vi "FolderMon Garbage Collector.vi"   [LabVIEW 2011]
uses:
  ITK EXT/utils/strutil.llb/Case Matching.ctl
  Summitek EXT/OpenG EXT/file/file.llb/File Exists - Scalar__ogtk.vi
  server lib/Spartan CONFIG Global.vi
types:
  T1 = typedef "Case Matching.ctl" = enum16{"a != A", "a == A", "system"}
  T2 = typedef "Keyed Array.ctl" = cluster{"keys":string[], "values":string[]}
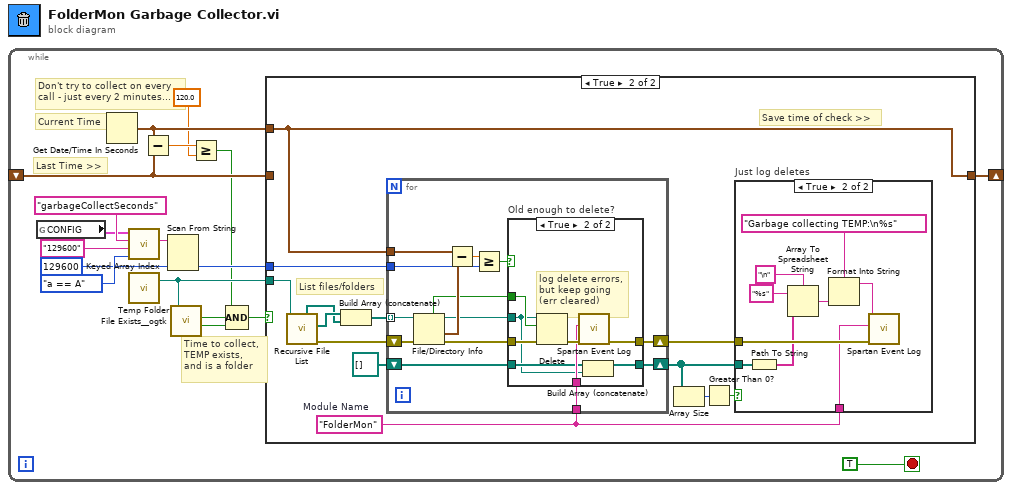
[diagram p0: block diagram]
diagram:
  n1 = while {
    shift-right: [w10] -> _
    shift-left: _ -> [w6]
    stop <- TRUE stop-if-true
    # "Time to collect,\nTEMP exists,\nand is a folder"
    # "Don't try to collect on every\ncall - just every 2 minutes..."
    # "Last Time >>"
    # "Current Time"
    n2 = global read "Spartan CONFIG Global.vi" "CONFIG"() -> (w14:T2)
    n3 = Get Date/Time In Seconds() -> (seconds since 1Jan1904=w7:timestamp)
    n4 = call "Keyed Array Index.vi"("case matching (sensitive)"=Case_Matching."a == A", "default value"="129600", "key"="garbageCollectSeconds", "array in"=w14) -> ("value"=w13:string)  [unwired: 3 out]
    n5 = call "Temp Folder.vi"() -> ("Temp Folder"=w18:path)  [unwired: 3 in]
    n6 = Subtract(x=w7, y=w6) -> (x-y=w8:dbl)
    n7 = Scan From String(input string=w13, default 1=129600) -> (output 1=w11:i32)  [unwired: 3 in, 3 out]
    n8 = call-poly "File Exists__ogtk.vi"("file path"=w18) -> ("is directory"=w3:bool, "exists"=w2:bool)  [unwired: 6 in]
    n9 = Greater Or Equal?(x=w8, y=120.0) -> (x >= y?=w4:bool)
    n10 = Compound Arithmetic op=AND(w4, w3, w2) -> (w1:bool)
    n11 = case shown="True" w1 {
      tunnel: w18 -> [_ w31]
      tunnel: w11 -> [_ w26]
      tunnel: w7 -> [_ w25]
      tunnel: [w19 w25] -> w10
      tunnel: w6 -> [w19 _]
      frame False {
      }
      frame True {
        w24 = "FolderMon"  # Module Name
        # "List files/folders"
        # "Save time of check >>"
        n12 = call <vilib>:"Recursive File List.vi"("Folder Path"=w31) -> ("error out"=w32:errorcluster, "All Files in Dir"=w30:path[], "All Folders"=w29:path[])  [unwired: 2 in, 6 out]
        n13 = Build Array (concatenate)(w30, w29) -> (w28:path[])
        n14 = for {
          shift-right: [w52] -> w27
          shift-left: w32 -> [w55]
          tunnel: w28 -> [w53] mode=indexing
          tunnel: w25 -> [w54]
          tunnel: w26 -> [w45]
          shift-right: [w43] -> w21
          shift-left: path[] [] ("appended array") -> [w44]
          tunnel: w24 -> [w42]
          n15 = File/Directory Info(path=w53, error in=w55) -> (path out=w49:path, directory=w46:bool, last mod=w51:timestamp, error out=w48:errorcluster)  [unwired: 3 out]
          n16 = Subtract(x=w54, y=w51) -> (x-y=w50:dbl)
          n17 = Greater Or Equal?(x=w50, y=w45) -> (x >= y?=w47:bool)
          n18 = case "Old enough to delete?" shown="True" w47 {
            tunnel: w49 -> [_ w58]
            tunnel: w48 -> [w57 w65]
            tunnel: [w57 w62] -> w52
            tunnel: w46 -> [_ w64]
            tunnel: w44 -> [w56 w60]
            tunnel: [w56 w59] -> w43
            tunnel: w42 -> [_ w61]
            frame False {
            }
            frame True {
              # "log delete errors,\nbut keep going\n(err cleared)"
              n19 = Delete(path (use dialog)=w58, entire hierarchy (F)=w64, error in=w65) -> (error out=w63:errorcluster)  [unwired: 4 out]
              n20 = call "Spartan Event Log.vi"("error in (no error)"=w63, "module (\"\")"=w61) -> ("error out"=w62:errorcluster)  [unwired: 3 in, 3 out]
              n21 = Build Array (concatenate)(w60, w58) -> (w59:path[])
            }
          }
        }
        n22 = Array Size(array=w21) -> (size(s)=w20:i32)
        n23 = Greater Than 0?(x=w20) -> (x > 0?=w23:bool)
        n24 = case "Just log deletes" shown="True" w23 {
          tunnel: w27 -> [_ w39]
          tunnel: w21 -> [_ w37]
          tunnel: w24 -> [_ w38]
          frame False {
          }
          frame True {
            n25 = Path To String(path=w37) -> (string=w36:string[])
            n26 = Array To Spreadsheet String(delimiter (Tab)="\n", array=w36, 3:"%s" ("delimiter (Tab)")) -> (spreadsheet string=w33:string)
            n27 = Format Into String(format string="Garbage collecting TEMP:\n%s" ("name (unnamed)"), w33) -> (resulting string=w40:string)  [unwired: 2 in, 1 out]
            n28 = call "Spartan Event Log.vi"("error in (no error)"=w39, "module (\"\")"=w38, "message (\"\")"=w40) -> ()  [unwired: 2 in, 4 out]
          }
        }
      }
    }
  }
